vi "Temperature Monitor.vi"() -> ()   [LabVIEW 2017]
doc: "This VI is the solution to an exercise in the LabVIEW Core 1 course.\n\nIt uses a While Loop and shift registers to average data. No hardware is necessary."
panel:
  in  "Stop Button":bool
  out "Temperature History":dbl(graph)
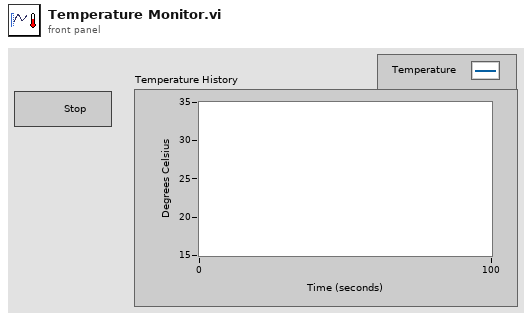
[diagram p1: front panel]
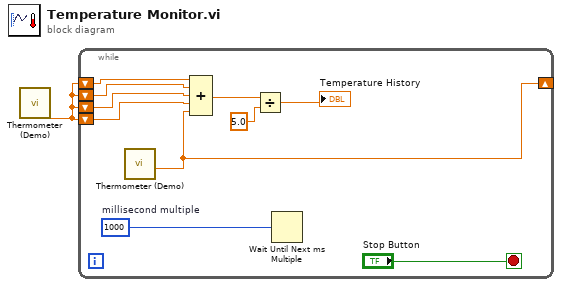
[diagram p0: block diagram]
diagram:
  n1 = call "Thermometer (Demo).vi"() -> ("Temperature Value"=w1:dbl)  [unwired: 11 in]
  n2 = while {
    shift-right: [w5] -> _
    shift-left: w1 -> [w9]
    shift-left: w1 -> [w8]
    shift-left: w1 -> [w7]
    shift-left: w1 -> [w6]
    stop <- "Stop Button" stop-if-true
    w11 = u32 1000  # millisecond multiple
    n3 = call "Thermometer (Demo).vi"() -> ("Temperature Value"=w5:dbl)  [unwired: 11 in]
    n4 = Compound Arithmetic op=ADD(w9, w8, w7, w6, w5) -> (w4:dbl)
    n5 = Divide(x=w4, y=5.0) -> (x/y=→"Temperature History":dbl)
    n6 = Wait Until Next ms Multiple(millisecond multiple=w11) -> ()  [unwired: 1 out]
  }
